vi "FP_Remove Scroll Bars while running.vi"(8 "Error":errorcluster, 11 "VI":refnum<vi>) -> (0 "Error Out":errorcluster, 3 "VI Out":refnum<vi>)   [LabVIEW 2020]
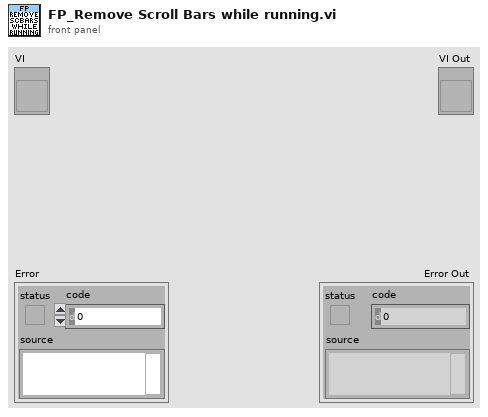
[diagram p1: front panel]
types:
  T1 = enum16{"Always On", "Always Off", "Off While Running"}
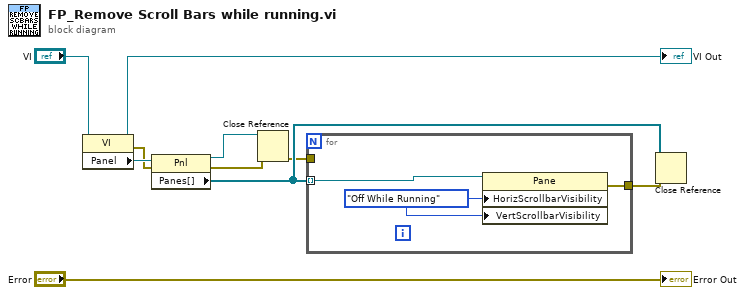
[diagram p0: block diagram]
diagram:
  n1 = property class="VI"(reference="VI") -> (reference out=→"VI Out":refnum<vi>, error out=w2:errorcluster, "Panel"=w7:refnum<vi>)  [unwired: 1 in]
  n2 = property class="Pnl"(reference=w7, error in=w2) -> (reference out=w6:refnum<vi>, error out=w3:errorcluster, "Panes[]"=w4:refnum<vi>[])
  n3 = Close Reference(reference=w6, error in (no error)=w3) -> (error out=w1:errorcluster)
  n4 = for {
    tunnel: w4 -> [w13] mode=indexing
    tunnel: [w11] -> w5
    tunnel: w1 -> [_]
    w12 = T1."Off While Running" ("Horizontal Scrollbar Visibility")
    n5 = property class="Pane"(reference=w13, "HorizScrollbarVisibility"=w12, "VertScrollbarVisibility"=w12) -> (error out=w11:errorcluster)  [unwired: 1 in, 1 out]
  }
  n6 = Close Reference(reference=w4, error in (no error)=w5) -> ()  [unwired: 1 out]
  "Error Out" <- "Error"
